vi "Tree.vi"() -> ()   [LabVIEW 2023]
doc: "Demonstrates the use of the Tree control."
panel:
  out "Multiple Selection Display Text":string[](array[string])
  out "Multiple Selection Value (tags)":string[](array[string])
  in  "Multiple Selection Tree":string[](tree)=["tag_item2", "tag_item3"]
  out "Single Selection Display Text":string
  out "Single Selection Value (tag)":string
  in  "Single Selection Tree":string(tree)="tag_item1"
  # "Overview: Demonstrates the use of the Tree control.\nInstructions:\n1. Select an item in the Single Selection Tree.\n2. Select multiple items in the Multiple Selection Tree by Ctrl-clicking the items (or Cmd-clicking on Mac OS).\n3. Run the VI. The values (tags) and display text of the selected items are displayed."
  # "To modify the item tags on a tree control, right-click on the Tree and select Edit Items. The display text can contain duplicates, but the item tags must be unique."
  # "To change the tree selection mode, right-click on the tree and change the Selection Mode."
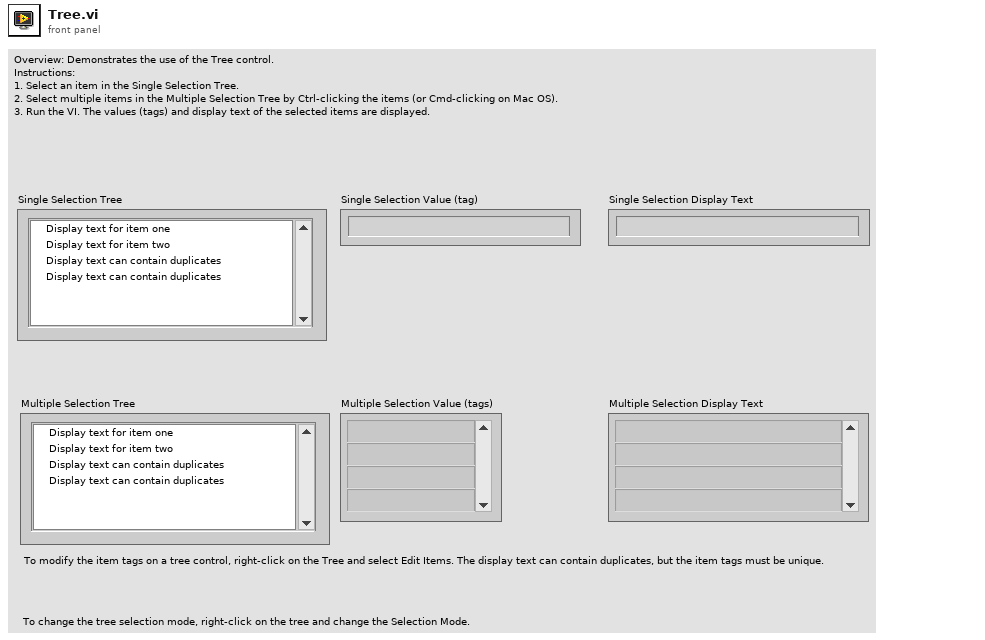
[diagram p1: front panel]
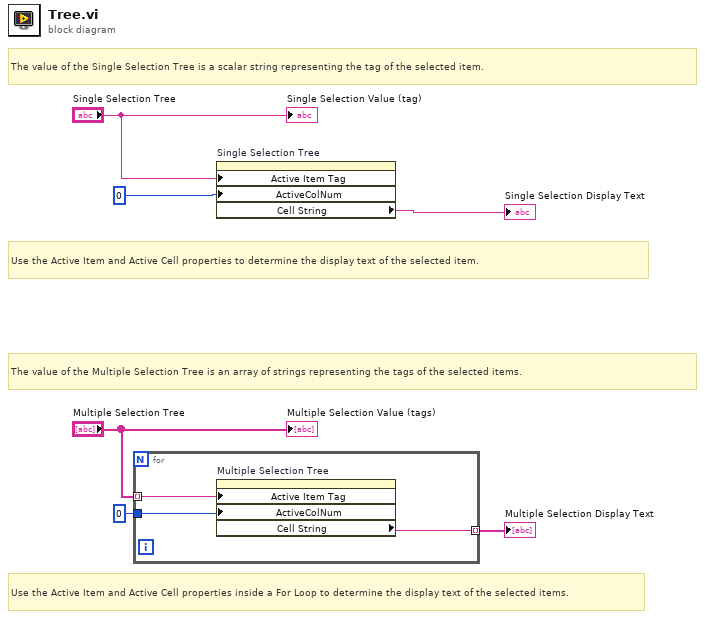
[diagram p0: block diagram]
diagram:
  # "The value of the Multiple Selection Tree is an array of strings representing the tags of the selected items."
  # "Use the Active Item and Active Cell properties inside a For Loop to determine the display text of the selected items."
  # "Use the Active Item and Active Cell properties to determine the display text of the selected item."
  # "The value of the Single Selection Tree is a scalar string representing the tag of the selected item."
  n1 = for {
    tunnel: 0 ("Active Cell:Active Column Number") -> [w9]
    tunnel: [w7] -> w3 mode=indexing
    tunnel: "Multiple Selection Tree" -> [w8] mode=indexing
    n2 = property on="Multiple Selection Tree" class="TreeControl (strict)"("Active Item Tag"=w8, "ActiveColNum"=w9) -> ("Cell String"=w7:string)  [unwired: 2 in, 2 out]
  }
  "Multiple Selection Display Text" <- w3
  n3 = property on="Single Selection Tree" class="TreeControl (strict)"("Active Item Tag"="Single Selection Tree", "ActiveColNum"=0 ("Active Cell:Active Column Number")) -> ("Cell String"=→"Single Selection Display Text":string)  [unwired: 2 in, 2 out]
  "Single Selection Value (tag)" <- "Single Selection Tree"
  "Multiple Selection Value (tags)" <- "Multiple Selection Tree"
